vi "save new device group.vi"(10 "ItemSyms in":i32[](array[numeric]), 11 "MulticolumnListbox in":refnum<vi>) -> (0 "error out":errorcluster, 3 "ItemSyms out":i32[](array[numeric]))   [LabVIEW 2020]
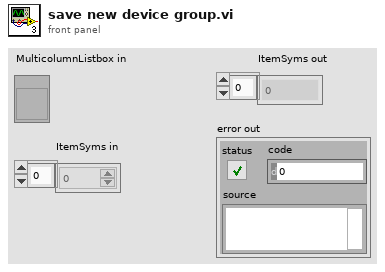
[diagram p1: front panel]
types:
  T1 = typedef "mysql_authentication.ctl" = cluster{"User":string, "Password":string, "Database":string}
  T2 = cluster{"Port":u16, "IP Address":string, "Authentication":T1}
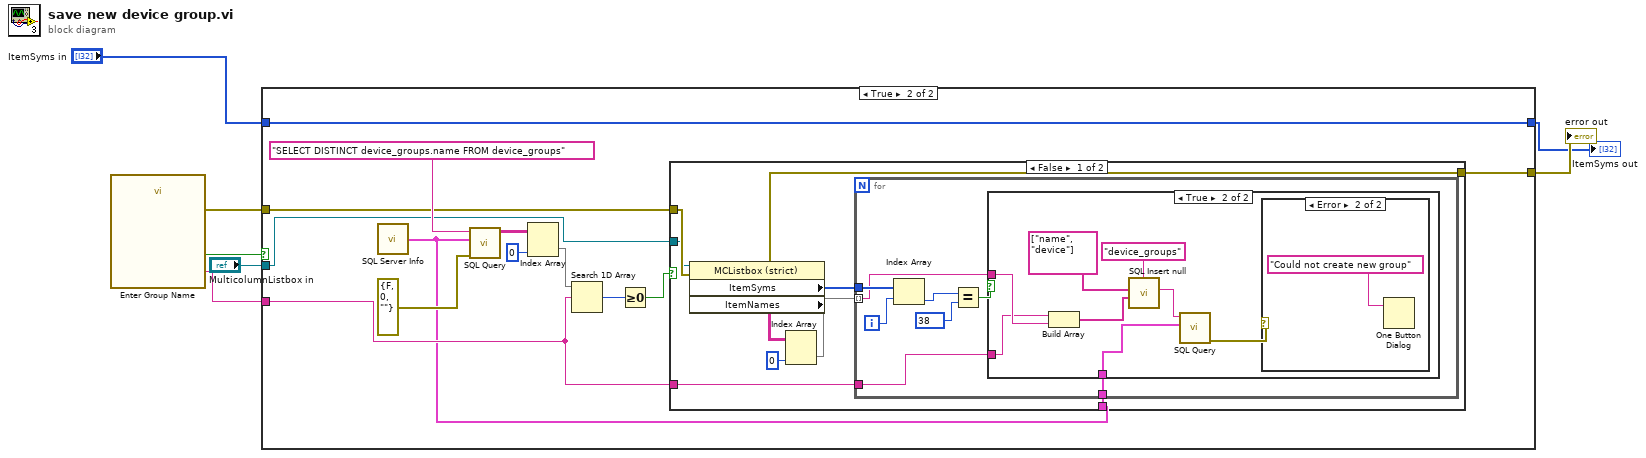
[diagram p0: block diagram]
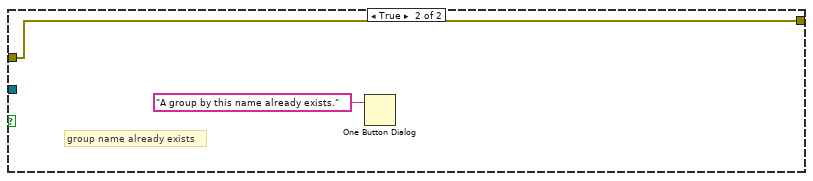
[diagram p5: hidden frame]
diagram:
  n1 = call "Enter Group Name"() -> ("Group Name"=w3:string, "Create Group"=w2:bool, "error out"=w6:errorcluster)  [unwired: 17 in]
  n2 = case shown="True" w2 {
    tunnel: w3 -> [_ w15]
    tunnel: "ItemSyms in" -> [w9 w14]
    tunnel: [w9 w14] -> w5
    tunnel: w6 -> [w8 w13]
    tunnel: [w8 w12] -> w7
    tunnel: "MulticolumnListbox in" -> [_ w10]
    frame False {
    }
    frame True {
      n3 = call "SQL Server Info.vi"() -> ("SQL Server Info"=w11:T2)
      n4 = call "SQL Query.vi"("error in (no error)"=errorcluster {"status"=FALSE, "code"=0, "source"=""}, "SQL Server Info"=w11, "Query"="SELECT DISTINCT device_groups.name FROM device_groups") -> ("data"=w20:string[][])  [unwired: 7 in, 1 out]
      n5 = Index Array(array=w20, index (col)=0 ("disabled index (col)")) -> (element=w18:string[])  [unwired: 1 in]
      n6 = Search 1D Array(1D array=w18, element=w15) -> (index of element=w17:i32)  [unwired: 1 in]
      n7 = Greater Or Equal To 0?(x=w17) -> (x >= 0?=w16:bool)
      n8 = case shown="False" w16 {
        tunnel: w15 -> [w27 _]
        tunnel: w13 -> [w26 w49]
        tunnel: [w25 w49] -> w12
        tunnel: w11 -> [w24 _]
        tunnel: w10 -> [w23 _]
        frame False {
          n9 = property on="Property Node" class="MCListbox (strict)"(reference=w23, error in=w26) -> (error out=w25:errorcluster, "ItemSyms"=w29:i32[], "ItemNames"=w30:string[][])  [unwired: 1 out]
          n10 = Index Array(array=w30, index (col)=0 ("disabled index (col)")) -> (element=w28:string[])  [unwired: 1 in]
          n11 = for {
            tunnel: w28 -> [w34] mode=indexing
            tunnel: w29 -> [w38]
            tunnel: w27 -> [w33]
            tunnel: w24 -> [w32]
            i -> [w36]
            n12 = Index Array(array=w38, index=w36) -> (element=w37:i32)
            n13 = Equal?(x=w37, y=38) -> (x = y?=w35:bool)
            n14 = case shown="True" w35 {
              tunnel: w34 -> [_ w44]
              tunnel: w33 -> [_ w43]
              tunnel: w32 -> [_ w40]
              frame False {
              }
              frame True {
                n15 = Build Array(w43, w44) -> (w47:string[])
                n16 = call "SQL Insert null.vi"("Values"=w47, "Column Names"=string[] ["name", "device"] ("appended array"), "Table"="device_groups") -> ("Query String"=w42:string)  [unwired: 8 in]
                n17 = call "SQL Query.vi"("SQL Server Info"=w40, "Query"=w42) -> ("error out"=w41:errorcluster)  [unwired: 8 in, 1 out]
                n18 = case shown="Error" w41 {
                  frame No Error {
                  }
                  frame Error {
                    n19 = One Button Dialog(message="Could not create new group") -> ()  [unwired: 1 in, 1 out]
                  }
                }
              }
            }
          }
        }
        frame True {
          # "group name already exists"
          n20 = One Button Dialog(message="A group by this name already exists.") -> ()  [unwired: 1 in, 1 out]
        }
      }
    }
  }
  "error out" <- w7
  "ItemSyms out" <- w5
